vi "Call Vi.vi"(7 "Auto Dispose Ref":bool, 8 "error in (no error)":errorcluster caption="错误输入（无错误）", 10 "Vi Path":path, 11 "PanelDataNode 输入":refnum<class "PanelDataNode.lvclass">) -> (0 "error out":errorcluster caption="错误输出", 2 "VI*":refnum<vi>, 3 "PanelDataNode 输出":refnum<class "PanelDataNode.lvclass">)   [LabVIEW 2013, in "PanelDataNode.lvclass"]
uses:
  PanelDataNode.lvclass
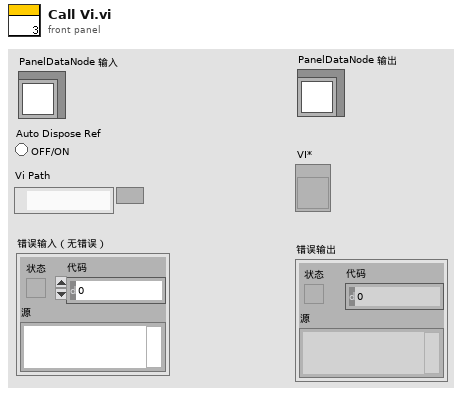
[diagram p1: front panel]
types:
  T1 = enum32{"Bad", "Idle", "Run top level", "Running"}
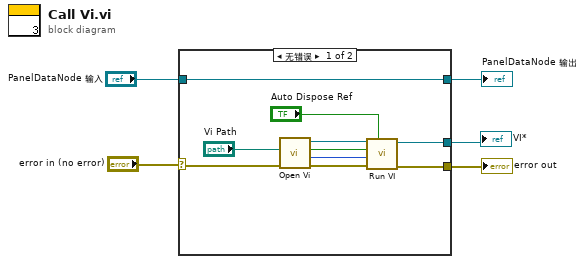
[diagram p0: block diagram]
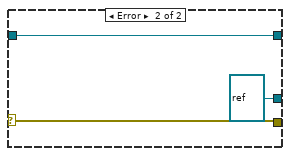
[diagram p2: hidden frame]
diagram:
  n1 = case shown="无错误" "error in (no error)" {
    selector: "error in (no error)" -> [w11 w18]
    tunnel: [w12 w18] -> w5
    tunnel: "PanelDataNode 输入" -> [w10 w17]
    tunnel: [w10 w17] -> w2
    tunnel: [w7 refnum<vi> refnum ("VI*")] -> w1
    frame No Error {
      n2 = call "Open Vi.vi"("error in (no error)"=w11, "Vi Path"="Vi Path") -> ("error out"=w13:errorcluster, "Exec.State"=w8:T1, "IsCloneVI"=w9:bool, "VI*"=w14:refnum<vi>)  [unwired: 6 in]
      n3 = call "Run VI.vi"("Auto Dispose Ref"="Auto Dispose Ref", "error in (no error)"=w13, "Exec.State"=w8, "clone vi?"=w9, "VI*"=w14) -> ("error out"=w12:errorcluster, "VI*"=w7:refnum<vi>)  [unwired: 5 in]
    }
    frame Error {
    }
  }
  "PanelDataNode 输出" <- w2
  "error out" <- w5
  "VI*" <- w1
